vi "Main UI.vi"(8 "error in (no error)":errorcluster, 10 "Initial Mouse (Demo)":refnum<class "Mouse.lvclass">) -> (0 "error out":errorcluster)   [LabVIEW 2020, in "App.lvlib" / "MazeUI.lvclass"]
uses:
  MazeUI.lvclass
  Maze/Maze/Maze.lvclass
  Maze/Mouse/Mouse.lvclass
  Mouse Type.ctl
  Maze/Direction.ctl
  <vilib>/Platform/browser.llb/Open URL in Default Browser (string).vi
  <vilib>/Utility/cursorutil.llb/Set Cursor (Icon Pict).vi
  Help UI.vi
  <vilib>/regexp/Match Regular Expression.xnode
  MazeFileIO/MazeFileIO.lvclass
  Maze/Maze.lvlib
  Maze/MazeGen/MazeGen.lvclass
panel:
  in  "Help Button":bool
  in  "Forums":bool
  in  "Configure Mouse":bool
  out "Mouse Name":string="Demo Mouse"
  in  "Run Speed":i32(slide)=100 scale=500.0..0.5
  out "Stepping":bool
  in  "Reset":bool
  in  "Step":bool
  out "Path":picture
  out "Walls":picture
  out "Actions":i32
  out "Mouse":refnum<class "Mouse.lvclass">
  in  "Stop":bool
  out "Running":bool
  out "Maze":refnum<class "Maze.lvclass">
  in  "Save":bool
  in  "Random":bool
  out "Maze":string
  in  "Load Maze":bool
  out "Status":string
  out "Mouse Author":string="Demo Mouse"
  in  "Load Mouse":bool
  in  "Start":bool
  out "Display":picture
  # "Summer of LabVIEW Maze Challenge"
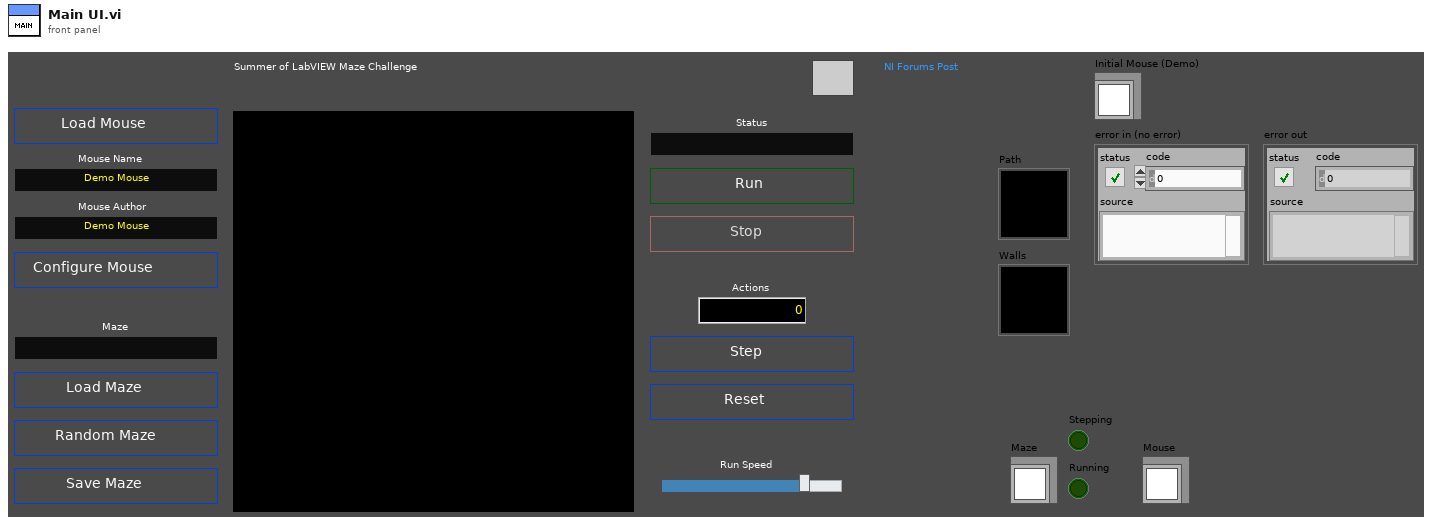
[diagram p1: front panel]
types:
  T1 = enum32{"Invalid", "Standard", "Closed", "Hidden", "Minimized", "Maximized"}
  T2 = enum8{"Enabled", "Disabled", "Disabled and Grayed Out"}
  T3 = typedef "App.lvlib/MazeUI.lvclass/Mouse Type.ctl" = enum16{"Instance", "Class Path", "LLB Path"}
  T4 = typedef "Maze.lvlib/Direction.ctl" = enum8{"East", "North", "West", "South"}
  T5 = typedef "Maze.lvlib/Position.ctl" = cluster{"S":i32, "E":i32}
  T6 = enum32{"Bad", "Idle", "Run top level", "Running"}
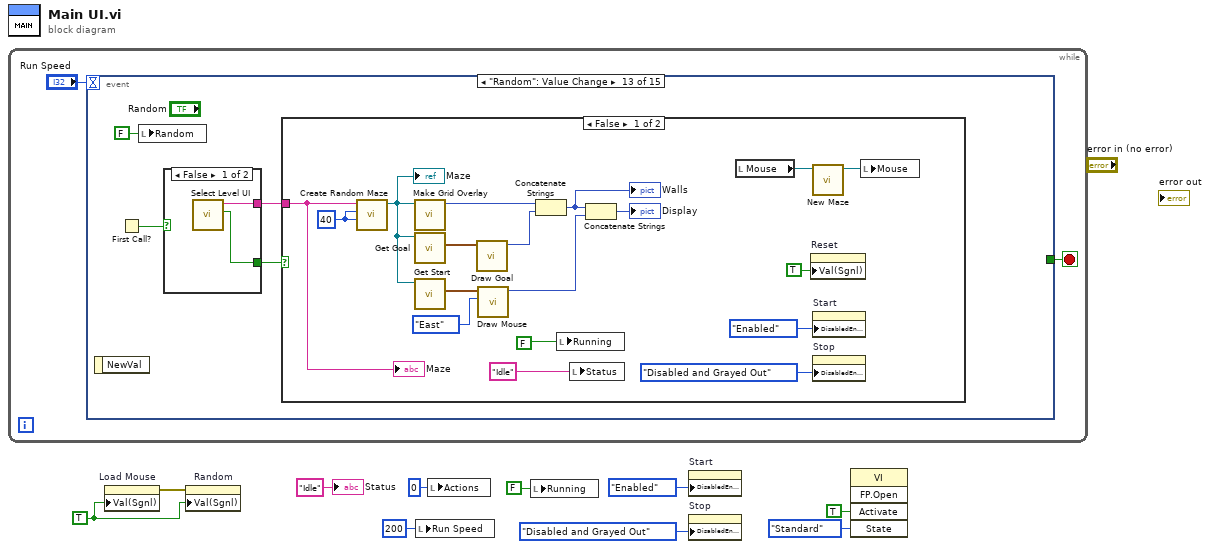
[diagram p0: block diagram]
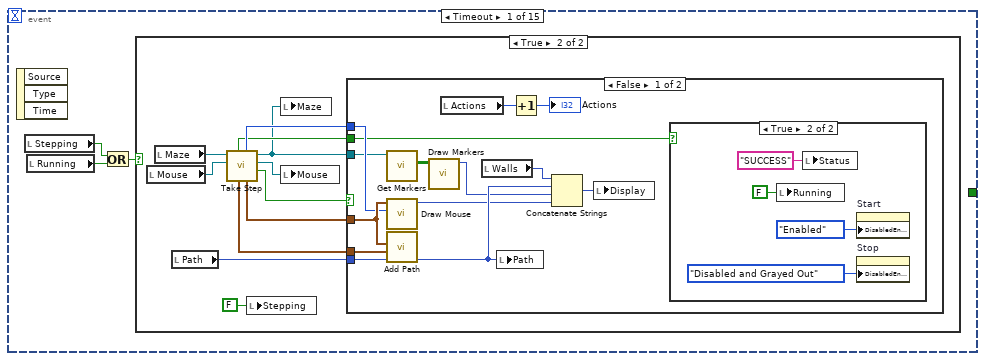
[diagram p2: hidden frame]
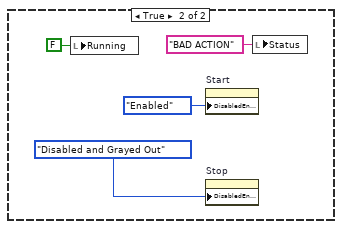
[diagram p5: hidden frame]
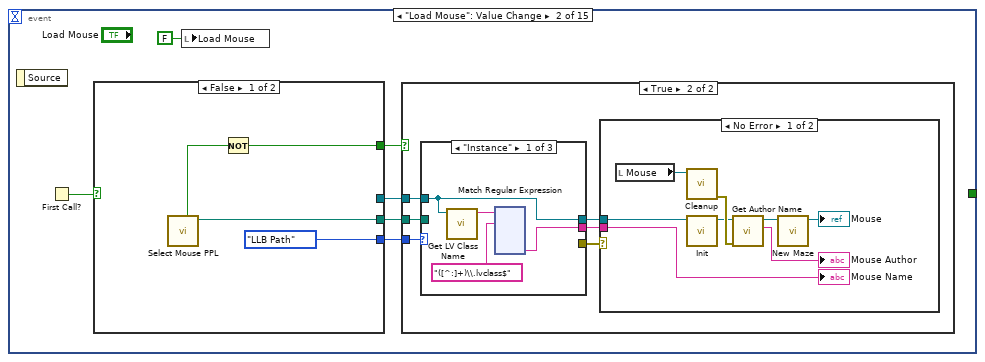
[diagram p6: hidden frame]
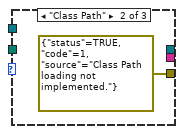
[diagram p8: hidden frame]
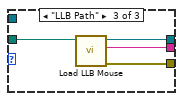
[diagram p9: hidden frame]
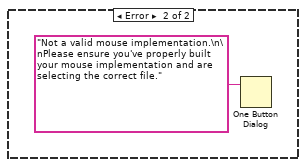
[diagram p10: hidden frame]
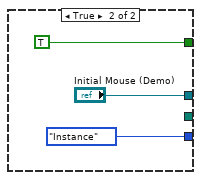
[diagram p11: hidden frame]
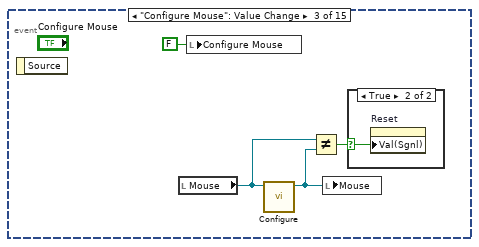
[diagram p12: hidden frame]
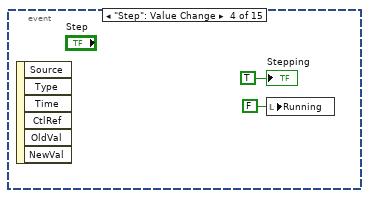
[diagram p14: hidden frame]
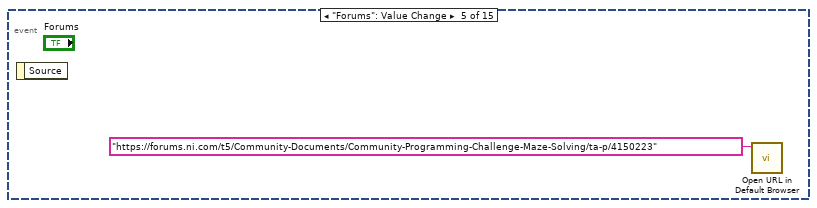
[diagram p15: hidden frame]
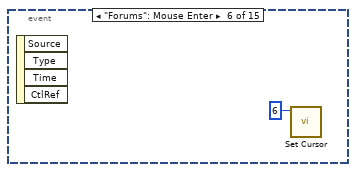
[diagram p16: hidden frame]
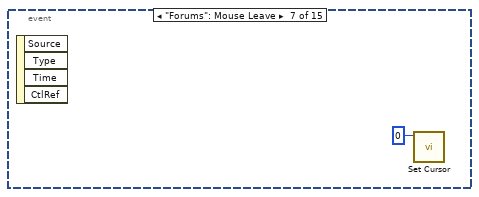
[diagram p17: hidden frame]
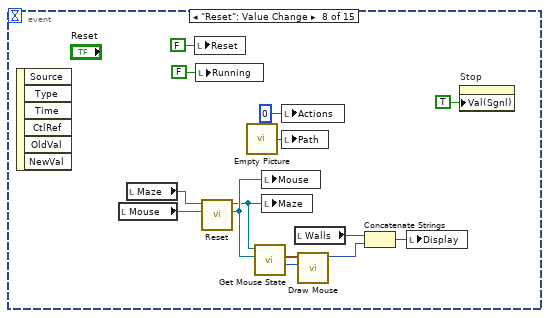
[diagram p18: hidden frame]
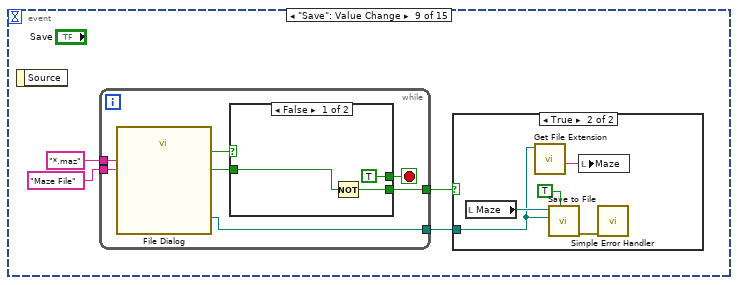
[diagram p19: hidden frame]
diagram:
  w4 = TRUE ("Value (Signaling)")
  n1 = while {
    stop <- w12 stop-if-true
    n2 = event shown="[12] \"Random\": Value Change" {
      selector: _ -> [_ _ _ _ _ _ _ _ _ _ _ _ _ _ _]
      dyn-events: _ -> [_ _ _ _ _ _ _ _ _ _ _ _ _ _ _]
      timeout: "Run Speed" -> [_ _ _ _ _ _ _ _ _ _ _ _ _ _ _]
      tunnel: [_ _ _ _ _ _ _ _ _ TRUE ("Discard?") _ _ _ _ _] -> w12
      event Timeout {
        n3 = event-data() -> ()  [unwired: 1 in, 3 out]
        n4 = local read "Stepping"() -> (w13:bool)
        n5 = local read "Running"() -> (w15:bool)
        n6 = Or(x=w13, y=w15) -> (x .or. y?=w14:bool)
        n7 = case shown="True" w14 {
          frame False {
          }
          frame True {
            n8 = local read "Mouse"() -> (w18:refnum<class "Mouse.lvclass">)
            n9 = local read "Maze"() -> (w26:refnum<class "Maze.lvclass">)
            n10 = local read "Path"() -> (w21:picture)
            n11 = call "Take Step.vi"("Mouse In"=w18, "Maze in"=w26) -> ("Bad Action?"=w25:bool, "Mouse"=w19:refnum<class "Mouse.lvclass">, "Maze"=w16:refnum<class "Maze.lvclass">, "New Position"=w23:T5, "Direction"=w24:T4, "Old Position"=w22:T5, "Goal?"=w17:bool)  [unwired: 2 in, 1 out]
            n12 = local write "Stepping"(FALSE ("Stepping")) -> ()
            n13 = local write "Maze"(w16) -> ()
            n14 = local write "Mouse"(w19) -> ()
            n15 = case shown="False" w25 {
              tunnel: w24 -> [w32 _]
              tunnel: w23 -> [w33 _]
              tunnel: w22 -> [w39 _]
              tunnel: w21 -> [w40 _]
              tunnel: w17 -> [w31 _]
              tunnel: w16 -> [w29 _]
              frame False {
                n16 = call "Get Markers.vi"("Maze in"=w29) -> ("Markers"=w28:bool[][])  [unwired: 8 in, 2 out]
                n17 = call "Draw Mouse.vi"("Direction"=w32, "Position"=w33) -> ("Picture"=w30:picture)  [unwired: 9 in]
                n18 = call "Add Path.vi"("Path In"=w40, "Old Position"=w39, "New Position"=w33) -> ("Path"=w37:picture)  [unwired: 8 in]
                n19 = call "Draw Markers.vi"("Markers"=w28) -> ("Picture"=w27:picture)  [unwired: 10 in]
                n20 = local read "Actions"() -> (w35:i32)
                n21 = local read "Walls"() -> (w38:picture)
                n22 = local write "Path"(w37) -> ()
                n23 = Increment(x=w35) -> (x+1=→"Actions":i32)
                n24 = Concatenate Strings(w38, w37, w27, w30) -> (w36:picture)
                n25 = local write "Display"(w36) -> ()
                n26 = case shown="True" w31 {
                  frame False {
                  }
                  frame True {
                    n27 = local write "Running"(FALSE ("Running")) -> ()
                    n28 = local write "Status"("SUCCESS" ("Status")) -> ()
                    n29 = property on="Start" class="Bool"("DisabledEnum"=T2."Enabled" ("Disabled")) -> ()  [unwired: 2 in, 2 out]
                    n30 = property on="Stop" class="Bool (strict)"("DisabledEnum"=T2."Disabled and Grayed Out" ("Disabled")) -> ()  [unwired: 2 in, 2 out]
                  }
                }
              }
              frame True {
                n31 = local write "Running"(FALSE ("Running")) -> ()
                n32 = property on="Start" class="Bool"("DisabledEnum"=T2."Enabled" ("Disabled")) -> ()  [unwired: 2 in, 2 out]
                n33 = property on="Stop" class="Bool (strict)"("DisabledEnum"=T2."Disabled and Grayed Out" ("Disabled")) -> ()  [unwired: 2 in, 2 out]
                n34 = local write "Status"("BAD ACTION" ("Status")) -> ()
              }
            }
          }
        }
      }
      event "Load Mouse": Value Change {
        n35 = event-data() -> ()  [unwired: 1 in, 1 out]
        n36 = First Call?() -> (First Call?: T/F=w53:bool)
        n37 = case shown="False" w53 {
          tunnel: [w196 TRUE] -> w52
          tunnel: [w198 _] -> w51
          tunnel: [Mouse_Type."LLB Path" ("Mouse Type") Mouse_Type."Instance" ("Mouse Type")] -> w50
          tunnel: [_ "Initial Mouse (Demo)"] -> w49
          frame False {
            n38 = call "Select Mouse PPL.vi"() -> ("selected path"=w198:path, "cancelled"=w197:bool)  [unwired: 10 in]
            n39 = Not(x=w197) -> (.not. x?=w196:bool)
          }
          frame True {
          }
        }
        n40 = local write "Load Mouse"(FALSE ("Load Mouse")) -> ()
        n41 = case shown="True" w52 {
          tunnel: w51 -> [_ w60]
          tunnel: w50 -> [_ w56]
          tunnel: w49 -> [_ w55]
          frame False {
          }
          frame True {
            n42 = case shown="\"Instance\"" w56 {
              tunnel: w60 -> [_ _ w185]
              tunnel: [w63 _ w184] -> w59
              tunnel: [w64 _ w183] -> w58
              tunnel: [_ errorcluster {"status"=TRUE, "code"=1, "source"="Class Path loading not implemented."} ("error out") w182] -> w57
              tunnel: w55 -> [w64 _ _]
              frame "Instance" {
                n43 = call <vilib>:"Get LV Class Name.vi"("object"=w64) -> ("class name"=w62:string)  [unwired: 9 in, 1 out]
                n44 = xnode "Match Regular Expression"("input string"=w62, "regular expression"="([^:]+)\\.lvclass$") -> ("submatch 1"=w63:string)  [unwired: 4 in, 5 out]
              }
              frame "Class Path" {
              }
              frame "LLB Path" {
                n45 = call "Load LLB Mouse.vi"("Mouse LLB"=w185) -> ("error out"=w182:errorcluster, "Name"=w184:string, "Mouse"=w183:refnum<class "Mouse.lvclass">)  [unwired: 8 in]
              }
            }
            n46 = case shown="No Error" w57 {
              tunnel: w58 -> [w189 _]
              tunnel: w59 -> [w188 _]
              frame No Error {
                n47 = local read "Mouse"() -> (w190:refnum<class "Mouse.lvclass">)
                n48 = call-dynamic "Cleanup.vi"("Mouse in"=w190) -> ("error out"=w193:errorcluster)  [unwired: 10 in]
                n49 = call-dynamic "Init.vi"("Mouse in"=w189) -> ("Mouse out"=w191:refnum<class "Mouse.lvclass">)  [unwired: 9 in, 1 out]
                n50 = call-dynamic "Get Author Name.vi"("error in (no error)"=w193, "Mouse in"=w191) -> ("Author"=→"Mouse Author":string, "Mouse out"=w187:refnum<class "Mouse.lvclass">)  [unwired: 7 in, 1 out]
                n51 = call-dynamic "New Maze.vi"("Mouse in"=w187) -> ("Mouse out"=→"Mouse":refnum<class "Mouse.lvclass">)  [unwired: 9 in, 1 out]
                "Mouse Name" <- w188
              }
              frame Error {
                n52 = One Button Dialog(message="Not a valid mouse implementation.\n\nPlease ensure you've properly built your mouse implementation and are selecting the correct file.") -> ()  [unwired: 1 in, 1 out]
              }
            }
          }
        }
      }
      event "Configure Mouse": Value Change {
        n53 = event-data() -> ()  [unwired: 1 in, 1 out]
        n54 = local read "Mouse"() -> (w203:refnum<class "Mouse.lvclass">)
        n55 = local write "Configure Mouse"(FALSE ("Configure Mouse")) -> ()
        n56 = call-dynamic "Configure.vi"("Mouse in"=w203) -> ("Mouse out"=w204:refnum<class "Mouse.lvclass">)  [unwired: 9 in, 1 out]
        n57 = Not Equal?(x=w203, y=w204) -> (x != y?=w202:bool)
        n58 = local write "Mouse"(w204) -> ()
        n59 = case shown="True" w202 {
          selector: w202 -> [_ w206]
          frame False {
          }
          frame True {
            n60 = property on="Reset" class="Bool (strict)"("Val(Sgnl)"=w206) -> ()  [unwired: 2 in, 2 out]
          }
        }
      }
      event "Step": Value Change {
        n61 = event-data() -> ()  [unwired: 1 in, 6 out]
        n62 = local write "Running"(FALSE ("Running")) -> ()
        "Stepping" <- TRUE ("Step")
      }
      event "Forums": Value Change {
        n63 = event-data() -> ()  [unwired: 1 in, 1 out]
        n64 = call-poly <vilib>:"Open URL in Default Browser.vi"("URL"="https://forums.ni.com/t5/Community-Documents/Community-Programming-Challenge-Maze-Solving/ta-p/4150223") -> ()  [unwired: 5 in, 2 out]
      }
      event "Forums": Mouse Enter {
        n65 = event-data() -> ()  [unwired: 1 in, 4 out]
        n66 = call-poly <vilib>:"Set Cursor.vi"("icon"=u16 6) -> ()  [unwired: 9 in, 2 out]
      }
      event "Forums": Mouse Leave {
        n67 = event-data() -> ()  [unwired: 1 in, 4 out]
        n68 = call-poly <vilib>:"Set Cursor.vi"("icon"=u16 0) -> ()  [unwired: 9 in, 2 out]
      }
      event "Reset": Value Change {
        n69 = event-data() -> ()  [unwired: 1 in, 6 out]
        n70 = local read "Mouse"() -> (w214:refnum<class "Mouse.lvclass">)
        n71 = local read "Maze"() -> (w224:refnum<class "Maze.lvclass">)
        n72 = local write "Reset"(FALSE ("Reset")) -> ()
        n73 = local write "Running"(FALSE ("Running")) -> ()
        n74 = call "Reset.vi"("Mouse In"=w214, "Maze in"=w224) -> ("Mouse"=w215:refnum<class "Mouse.lvclass">, "Maze out"=w213:refnum<class "Maze.lvclass">)  [unwired: 7 in, 1 out]
        n75 = call "Empty Picture"() -> ("empty picture"=w225:picture)
        n76 = call "Get Mouse State.vi"("Mouse"=w215, "Maze in"=w213) -> ("Direction"=w217:T4, "Position"=w218:T5)  [unwired: 6 in, 2 out]
        n77 = local write "Mouse"(w215) -> ()
        n78 = local write "Maze"(w213) -> ()
        n79 = local write "Actions"(0 ("Actions")) -> ()
        n80 = local write "Path"(w225) -> ()
        n81 = local read "Walls"() -> (w221:picture)
        n82 = call "Draw Mouse.vi"("Direction"=w217, "Position"=w218) -> ("Picture"=w220:picture)  [unwired: 9 in]
        n83 = Concatenate Strings(w221, w220) -> (w219:picture)
        n84 = local write "Display"(w219) -> ()
        n85 = property on="Stop" class="Bool (strict)"("Val(Sgnl)"=TRUE ("Value (Signaling)")) -> ()  [unwired: 2 in, 2 out]
      }
      event "Save": Value Change {
        n86 = event-data() -> ()  [unwired: 1 in, 1 out]
        n87 = while {
          tunnel: "*.maz" ("pattern (all files)") -> [w241]
          tunnel: "Maze File" ("pattern label") -> [w240]
          tunnel: [w237] -> w226
          tunnel: [w235] -> w227
          stop <- w236 stop-if-true
          n88 = call "File Dialog"("pattern (all files)"=w241, "pattern label"=w240) -> ("selected path"=w235:path, "exists"=w239:bool, "cancelled"=w238:bool)  [unwired: 10 in, 1 out]
          n89 = case shown="False" w239 {
            tunnel: w238 -> [w243 _]
            tunnel: [w244 w245] -> w237
            tunnel: [TRUE ("T button?") w245] -> w236
            frame False {
              n90 = Not(x=w243) -> (.not. x?=w244:bool)
            }
            frame True {
              n91 = Two Button Dialog(message="Are you sure you want to replace the file?", 2:"Yes" ("T button name (\"OK\")")) -> (T button?=w245:bool)  [unwired: 1 in]
            }
          }
        }
        n92 = case shown="True" w226 {
          tunnel: w227 -> [_ w231]
          frame False {
          }
          frame True {
            n93 = local read "Maze"() -> (w234:refnum<class "Maze.lvclass">)
            n94 = call <vilib>:"Get File Extension.vi"("file"=w231) -> ("filename without extension"=w230:string)  [unwired: 6 in, 4 out]
            n95 = call "Save to File.vi"("Replace if Exists? (F)"=TRUE, "Maze File Path (*.maz)"=w231, "Maze In"=w234) -> ("error out"=w232:errorcluster)  [unwired: 7 in, 1 out]
            n96 = local write "Maze"(w230) -> ()
            n97 = call <vilib>:"Simple Error Handler.vi"("error in (no error)"=w232) -> ()  [unwired: 4 in, 5 out]
          }
        }
      }
      event Panel Close {
        n98 = event-data() -> ()  [unwired: 1 in, 4 out]
        n99 = local read "Mouse"() -> (w248:refnum<class "Mouse.lvclass">)
        n100 = call-dynamic "Cleanup.vi"("Mouse in"=w248) -> ()  [unwired: 10 in, 1 out]
      }
      event "Help Button": Value Change {
        n101 = event-data() -> ()  [unwired: 1 in, 1 out]
        n102 = vi-ref "App.lvlib:MazeUI.lvclass:Help UI.vi"() -> (w255:refnum<vi>)
        n103 = property class="VI"(reference=w255) -> (reference out=w251:refnum<vi>, "Exec.State"=w254:T6)  [unwired: 1 in, 1 out]
        n104 = case shown="Default" w254 {
          tunnel: w251 -> [w256 w260]
          tunnel: [w256 w257] -> w250
          frame "Run top level", "Running" {
          }
          frame Default {
            n105 = invoke class="VI" method="Run VI"(reference=w260, "Wait until done"=FALSE ("Wait Until Done"), "Auto Dispose Ref"=TRUE ("Auto Dispose Reference")) -> (reference out=w257:refnum<vi>)  [unwired: 2 in, 4 out]
          }
        }
        n106 = invoke class="VI" method="FP.Open"(reference=w250, "Activate"=TRUE ("Activate?"), "State"=T1."Standard") -> ()  [unwired: 2 in, 5 out]
      }
      event "Load Maze": Value Change {
        n107 = event-data() -> ()  [unwired: 1 in, 1 out]
        n108 = call "File Dialog2"("pattern (all files)"="*.maz", "pattern label"="Maze File") -> ("selected path"=w264:path, "cancelled"=w261:bool)  [unwired: 10 in, 2 out]
        n109 = case shown="False" w261 {
          tunnel: w264 -> [w265 _]
          frame False {
            n110 = call "Load From File.vi"("Maze File Path (*.maz)"=w265) -> ("error out"=w266:errorcluster, "Maze"=w268:refnum<class "Maze.lvclass">)  [unwired: 9 in]
            n111 = case shown="No Error" w266 {
              selector: w266 -> [_ w278]
              tunnel: w268 -> [w273 _]
              tunnel: w265 -> [w272 _]
              frame No Error {
                n112 = local write "Maze"(w273) -> ()
                n113 = call <vilib>:"Get File Extension.vi"("file"=w272) -> ("filename without extension"=w271:string)  [unwired: 6 in, 4 out]
                n114 = call "Make Grid Overlay.vi"("Maze"=w273) -> ("Picture"=w276:picture)  [unwired: 10 in]
                n115 = call "Get Goal.vi"("Maze in"=w273) -> ("Goal"=w275:T5)  [unwired: 8 in, 2 out]
                n116 = call "Draw Goal.vi"("Position"=w275) -> ("Picture"=w274:picture)  [unwired: 10 in]
                n117 = local write "Maze"(w271) -> ()
                n118 = Concatenate Strings(w276, w274) -> (w277:picture)
                n119 = local read "Mouse"() -> (w270:refnum<class "Mouse.lvclass">)
                n120 = local write "Walls"(w277) -> ()
                n121 = call-dynamic "New Maze.vi"("Mouse in"=w270) -> ("Mouse out"=w269:refnum<class "Mouse.lvclass">)  [unwired: 9 in, 1 out]
                n122 = local write "Mouse"(w269) -> ()
              }
              frame Error {
                n123 = call <vilib>:"Simple Error Handler.vi"("error in (no error)"=w278) -> ()  [unwired: 4 in, 5 out]
              }
            }
            n124 = property on="Reset" class="Bool (strict)"("Val(Sgnl)"=TRUE ("Value (Signaling)")) -> ()  [unwired: 2 in, 2 out]
          }
          frame True {
          }
        }
      }
      event "Random": Value Change {
        n125 = event-data() -> ()  [unwired: 1 in, 1 out]
        n126 = First Call?() -> (First Call?: T/F=w279:bool)
        n127 = local write "Random"(FALSE ("Random")) -> ()
        n128 = case shown="False" w279 {
          tunnel: [w284 "Basic" ("Selected Level")] -> w281
          tunnel: [w283 FALSE ("Cancelled?")] -> w280
          frame False {
            n129 = call "Select Level UI.vi"() -> ("Cancelled?"=w283:bool, "Selected Level"=w284:string)  [unwired: 10 in]
          }
          frame True {
          }
        }
        n130 = case shown="False" w280 {
          tunnel: w281 -> [w287 _]
          frame False {
            w290 = 40 ("Height")
            n131 = call "Create Random Maze.vi"("Height (40)"=w290, "Width (40)"=w290, "Maze Level"=w287) -> ("Maze"=w291:refnum<class "Maze.lvclass">)  [unwired: 7 in, 1 out]
            "Maze" <- w291
            n132 = call "Make Grid Overlay.vi"("Maze"=w291) -> ("Picture"=w304:picture)  [unwired: 10 in]
            n133 = call "Get Goal.vi"("Maze in"=w291) -> ("Goal"=w301:T5)  [unwired: 8 in, 2 out]
            n134 = call "Get Start.vi"("Maze in"=w291) -> ("Start"=w303:T5)  [unwired: 8 in, 2 out]
            n135 = call "Draw Goal.vi"("Position"=w301) -> ("Picture"=w300:picture)  [unwired: 10 in]
            n136 = call "Draw Mouse.vi"("Direction"=Direction."East", "Position"=w303) -> ("Picture"=w297:picture)  [unwired: 9 in]
            n137 = Concatenate Strings(w304, w300) -> (w299:picture)
            "Walls" <- w299
            n138 = local write "Running"(FALSE ("Running")) -> ()
            n139 = local write "Status"("Idle" ("Status")) -> ()
            n140 = Concatenate Strings(w299, w297) -> (→"Display":picture)
            n141 = local read "Mouse"() -> (w289:refnum<class "Mouse.lvclass">)
            n142 = property on="Reset" class="Bool (strict)"("Val(Sgnl)"=TRUE ("Value (Signaling)")) -> ()  [unwired: 2 in, 2 out]
            n143 = call-dynamic "New Maze.vi"("Mouse in"=w289) -> ("Mouse out"=w288:refnum<class "Mouse.lvclass">)  [unwired: 9 in, 1 out]
            n144 = property on="Start" class="Bool"("DisabledEnum"=T2."Enabled" ("Disabled")) -> ()  [unwired: 2 in, 2 out]
            n145 = property on="Stop" class="Bool (strict)"("DisabledEnum"=T2."Disabled and Grayed Out" ("Disabled")) -> ()  [unwired: 2 in, 2 out]
            n146 = local write "Mouse"(w288) -> ()
            "Maze" <- w287
          }
          frame True {
          }
        }
      }
      event "Start": Value Change {
        n147 = event-data() -> ()  [unwired: 1 in, 1 out]
        n148 = local read "Mouse"() -> (w308:refnum<class "Mouse.lvclass">)
        n149 = local read "Maze"() -> (w309:refnum<class "Maze.lvclass">)
        n150 = call "Empty Picture"() -> ("empty picture"=→"Path":picture)
        n151 = call "Reset.vi"("Mouse In"=w308, "Maze in"=w309) -> ("Mouse"=w307:refnum<class "Mouse.lvclass">, "Maze out"=w305:refnum<class "Maze.lvclass">)  [unwired: 7 in, 1 out]
        n152 = local write "Status"("Running" ("Status")) -> ()
        n153 = call-dynamic "Start.vi"("Mouse in"=w307) -> ("Mouse out"=w306:refnum<class "Mouse.lvclass">)  [unwired: 9 in, 1 out]
        n154 = local write "Maze"(w305) -> ()
        n155 = local write "Actions"(0 ("Actions")) -> ()
        n156 = local write "Mouse"(w306) -> ()
        n157 = property on="Start" class="Bool"("DisabledEnum"=T2."Disabled and Grayed Out" ("Disabled")) -> ()  [unwired: 2 in, 2 out]
        n158 = property on="Stop" class="Bool (strict)"("DisabledEnum"=T2."Enabled" ("Disabled")) -> ()  [unwired: 2 in, 2 out]
        "Running" <- TRUE ("Running")
      }
      event "Stop": Value Change {
        n159 = event-data() -> ()  [unwired: 1 in, 6 out]
        n160 = local write "Stop"(FALSE ("Stop")) -> ()
        n161 = local write "Running"(FALSE ("Running")) -> ()
        n162 = local write "Status"("Idle" ("Status")) -> ()
        n163 = property on="Start" class="Bool"("DisabledEnum"=T2."Enabled" ("Disabled")) -> ()  [unwired: 2 in, 2 out]
        n164 = property on="Stop" class="Bool (strict)"("DisabledEnum"=T2."Disabled and Grayed Out" ("Disabled")) -> ()  [unwired: 2 in, 2 out]
      }
    }
  }
  n165 = property on="Load Mouse" class="Bool (strict)"("Val(Sgnl)"=w4) -> (error out=w3:errorcluster)  [unwired: 2 in, 1 out]
  n166 = property on="Random" class="Bool (strict)"(error in=w3, "Val(Sgnl)"=w4) -> ()  [unwired: 1 in, 2 out]
  n167 = local write "Run Speed"(200 ("Run Speed")) -> ()
  n168 = local write "Actions"(0 ("Actions")) -> ()
  n169 = local write "Running"(FALSE ("Running")) -> ()
  n170 = property on="Start" class="Bool"("DisabledEnum"=T2."Enabled" ("Disabled")) -> ()  [unwired: 2 in, 2 out]
  n171 = property on="Stop" class="Bool (strict)"("DisabledEnum"=T2."Disabled and Grayed Out" ("Disabled")) -> ()  [unwired: 2 in, 2 out]
  n172 = invoke class="VI" method="FP.Open"("Activate"=TRUE ("Activate?"), "State"=T1."Standard") -> ()  [unwired: 3 in, 5 out]
  "Status" <- "Idle" ("Status")
